vi "LV SPECTRUM STOP.vi"(8 "error in (no error)":errorcluster, 9 "Handle In":T1) -> (0 "error out":errorcluster, 1 "Handle Out":T1)   [LabVIEW 2021]
uses:
  SciSDK_Labview.lvlib
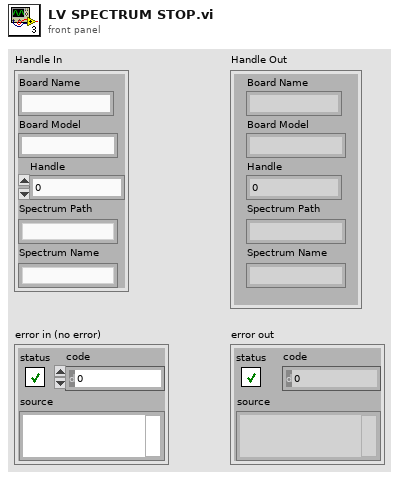
[diagram p1: front panel]
types:
  T1 = cluster{"Board Name":string, "Board Model":string, "Handle":u64, "Spectrum Path":string, "Spectrum Name":string}
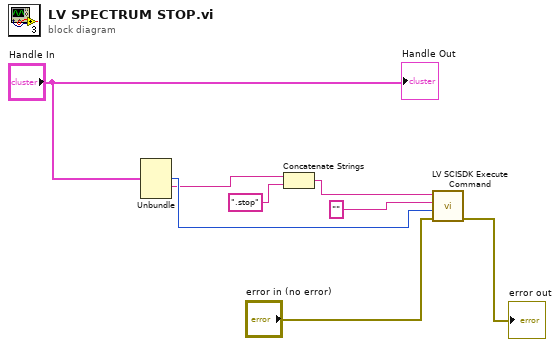
[diagram p0: block diagram]
diagram:
  n1 = Unbundle("Handle In") -> ("Handle"=w5:u64, "Spectrum Path"=w4:string)  [unwired: 3 out]
  n2 = Concatenate Strings(w4, ".stop" ("string")) -> (w7:string)
  n3 = call "LV SCISDK Execute Command.vi"("error in (no error)"="error in (no error)", "handle"=w5, "value"="", "Path"=w7) -> ("error out"=→"error out":errorcluster)  [unwired: 5 in, 2 out]
  "Handle Out" <- "Handle In"
